vi "Configure IQ Recorder Measurement Ratio.vi"(8 "error in (no error)":errorcluster, 9 "Ratio (1.0)":dbl=1.0 format="%^.3e", 10 "Instance (1)":i32=1, 11 "VISA resource name":refnum<visa-resource-name>) -> (0 "error out":errorcluster, 3 "VISA resource name out":refnum<visa-resource-name>)   [LabVIEW 2020, in "Rohde&Schwarz CMXP GPRF.lvlib"]
doc: "Reduces the sampling rate (as defined by the filter settings) by a factor <= 1 and thus extends the total measurement time.\n\nAttribute:\nRSCMXPGPRF_ATTR_IQ_RECORDER_MEASUREMENT_RATIO\n\nRemote-control command:\nCONFigure:GPRF:MEAS<i>:IQRecorder:RATio"
uses:
  <instrlib>/Rohde&Schwarz CMXP GPRF/Rohde&Schwarz CMXP GPRF.lvlib
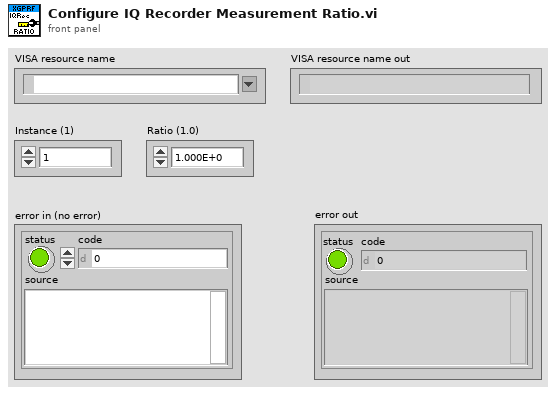
[diagram p1: front panel]
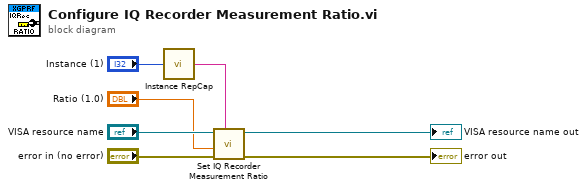
[diagram p0: block diagram]
diagram:
  n1 = call <instrlib>:"Instance RepCap.vi"("Instance in"="Instance (1)") -> ("Instance out"=w6:string)
  n2 = call "Set IQ Recorder Measurement Ratio"("Repeated Capabilities"=w6, "error in (no error)"="error in (no error)", "IQ Recorder Measurement Ratio (0.0)"="Ratio (1.0)", "instrument handle"="VISA resource name") -> ("error out"=→"error out":errorcluster, "instrument handle out"=→"VISA resource name out":refnum<visa-resource-name>)  [unwired: 6 in]
